vi "NXT_HINDBRAIN Write Data To Screen_01.vi"(7 "Clear Screen?":bool, 8 "Battery Voltage (mV)":u32, 9 "_irServoData":T1, 10 "_irData":T3, 11 "NXT":T2) -> ()   [LabVIEW 2012]
uses:
  irData_t.ctl
  <vilib>/NXT/Subs/LVHSConnector.ctl
  irServoData_t.ctl
  <vilib>/NXT/Dual Mode Library/Display/drawText.vi
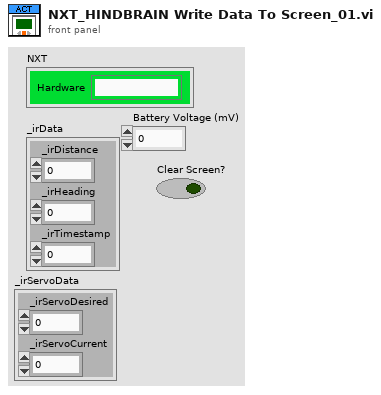
[diagram p1: front panel]
types:
  T1 = typedef "irServoData_t.ctl" = cluster{"_irServoDesired":i16, "_irServoCurrent":i16}
  T2 = typedef "LVHSConnector.ctl" = cluster{"Hardware":string, "Flattened String":string}
  T3 = typedef "irData_t.ctl" = cluster{"_irDistance":i32, "_irHeading":i32, "_irTimestamp":u32}
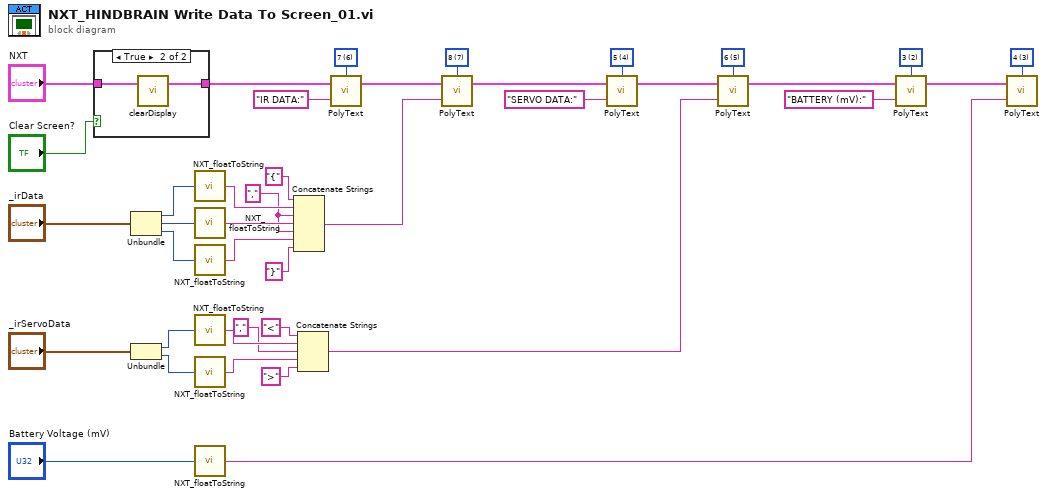
[diagram p0: block diagram]
diagram:
  w5 = i16 3 items=["1", "2", "3", "4", "5", "6", "7", "8"] ("Line")
  w7 = i16 2 items=["1", "2", "3", "4", "5", "6", "7", "8"] ("Line")
  w19 = i16 5 items=["1", "2", "3", "4", "5", "6", "7", "8"] ("Line")
  w21 = i16 4 items=["1", "2", "3", "4", "5", "6", "7", "8"] ("Line")
  w24 = i16 7 items=["1", "2", "3", "4", "5", "6", "7", "8"] ("Line")
  w26 = "," ("string")
  w35 = i16 6 items=["1", "2", "3", "4", "5", "6", "7", "8"] ("Line")
  n1 = case shown="True" "Clear Screen?" {
    tunnel: "NXT" -> [w40 w42]
    tunnel: [w40 w41] -> w36
    frame False {
    }
    frame True {
      n2 = call <vilib>:"clearDisplay.vi"("NXT"=w42) -> ("NXT"=w41:T2)  [unwired: 3 in]
    }
  }
  n3 = Unbundle("_irData") -> ("_irDistance"=w33:i32, "_irHeading"=w32:i32, "_irTimestamp"=w31:u32)
  n4 = Unbundle("_irServoData") -> ("_irServoDesired"=w14:i16, "_irServoCurrent"=w15:i16)
  n5 = call <vilib>:"NXT_floatToString.vi"("number"=w33) -> ("string"=w29:string)
  n6 = call <vilib>:"NXT_floatToString.vi"("number"=w32) -> ("string"=w28:string)
  n7 = call <vilib>:"NXT_floatToString.vi"("number"=w31) -> ("string"=w27:string)
  n8 = call <vilib>:"NXT_floatToString.vi"("number"=w14) -> ("string"=w13:string)
  n9 = call <vilib>:"NXT_floatToString.vi"("number"=w15) -> ("string"=w12:string)
  n10 = call <vilib>:"NXT_floatToString.vi"("number"="Battery Voltage (mV)") -> ("string"=w1:string)
  n11 = Concatenate Strings("{" ("string"), w29, w26, w28, w26, w27, "}" ("string")) -> (w22:string)
  n12 = Concatenate Strings("<" ("string"), w13, "," ("string"), w12, ">" ("string")) -> (w8:string)
  n13 = call-poly <vilib>:"PolyText.vi"("Text"="IR DATA:", "NXT"=w36, "Line"=w35) -> ("NXT"=w23:T2)  [unwired: 1 in]
  n14 = call-poly <vilib>:"PolyText.vi"("Text"=w22, "NXT"=w23, "Line"=w24) -> ("NXT"=w17:T2)  [unwired: 1 in]
  n15 = call-poly <vilib>:"PolyText.vi"("Text"="SERVO DATA:", "NXT"=w17, "Line"=w21) -> ("NXT"=w18:T2)  [unwired: 1 in]
  n16 = call-poly <vilib>:"PolyText.vi"("Text"=w8, "NXT"=w18, "Line"=w19) -> ("NXT"=w3:T2)  [unwired: 1 in]
  n17 = call-poly <vilib>:"PolyText.vi"("Text"="BATTERY (mV):", "NXT"=w3, "Line"=w7) -> ("NXT"=w4:T2)  [unwired: 1 in]
  n18 = call-poly <vilib>:"PolyText.vi"("Text"=w1, "NXT"=w4, "Line"=w5) -> ()  [unwired: 1 in, 1 out]
